vi "Try Parse.vi"(0 "SA Path in":refnum<class "SA 18GHz Path.lvclass">, 5 "Config Row":string[](array[string]), 11 "error in":errorcluster) -> (4 "SA Path out":refnum<class "SA 18GHz Path.lvclass">, 6 "Is of type?":bool=TRUE, 15 "error out":errorcluster)   [LabVIEW 2023, in "RFFixtureCharact.RFPM.lvlib" / "SA 18GHz Path.lvclass"]
uses:
  SA 18GHz Path.lvclass
  Common/RFCalAndFixtureCharact.Common.lvlib
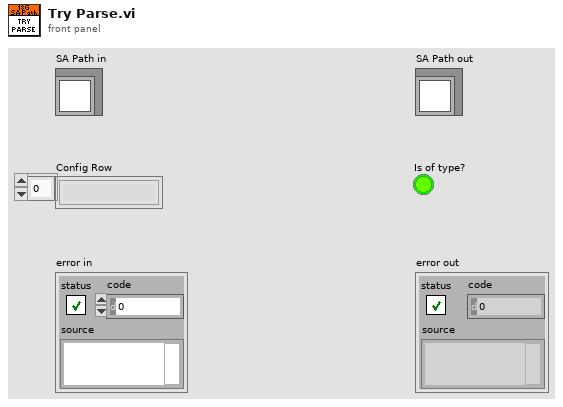
[diagram p1: front panel]
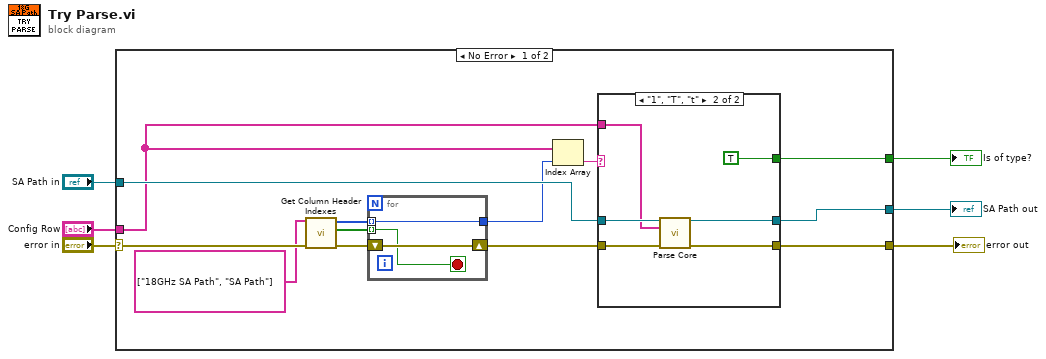
[diagram p0: block diagram]
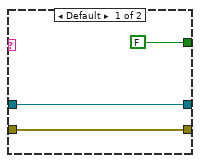
[diagram p2: hidden frame]
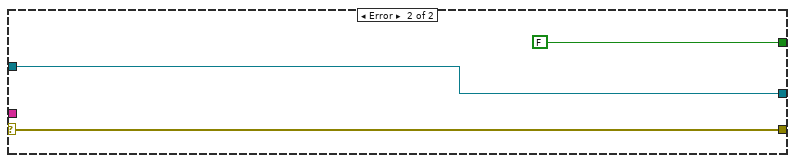
[diagram p3: hidden frame]
diagram:
  n1 = case shown="No Error" "error in" {
    selector: "error in" -> [w18 w34]
    tunnel: [w12 w34] -> w1
    tunnel: [w19 FALSE ("Is of type?")] -> w2
    tunnel: [w13 w33] -> w3
    tunnel: "Config Row" -> [w16 _]
    tunnel: "SA Path in" -> [w17 w33]
    frame No Error {
      n2 = call "Get Column Header Indexes.vi"("Column Header Names"=string[] ["18GHz SA Path", "SA Path"], "error in"=w18) -> ("Column Header Indices"=w11:i32[], "Column Header Exists?"=w10:bool[], "error out"=w9:errorcluster)  [unwired: 11 in]
      n3 = for {
        tunnel: w11 -> [w20] mode=indexing
        tunnel: w10 -> [w21] mode=indexing
        shift-right: [w22] -> w8
        shift-left: w9 -> [w22]
        tunnel: [w20] -> w7
        stop <- w21 stop-if-true
      }
      n4 = Index Array(array=w16, index=w7) -> (element=w15:string)
      n5 = case shown="\"1\", \"T\", \"t\"" w15 {
        tunnel: [w23 w31] -> w12
        tunnel: [FALSE ("Is of type?") TRUE ("Is of type?")] -> w19
        tunnel: [w25 w26] -> w13
        tunnel: w8 -> [w23 w30]
        tunnel: w17 -> [w25 w29]
        tunnel: w16 -> [_ w28]
        frame Default {
        }
        frame "1", "T", "t" {
          n6 = call-dynamic "Parse Core.vi"("SA Path in"=w29, "Config Row"=w28, "error in"=w30) -> ("SA Path out"=w26:refnum<class "SA 18GHz Path.lvclass">, "error out"=w31:errorcluster)  [unwired: 11 in]
        }
      }
    }
    frame Error {
    }
  }
  "error out" <- w1
  "SA Path out" <- w3
  "Is of type?" <- w2
